vi "PSU_VOUT_Converter.vi"(0 "Output %":dbl) -> (1 "decimal integer string":string, 2 "Output % duplicate":dbl)   [LabVIEW 2022 SP3]
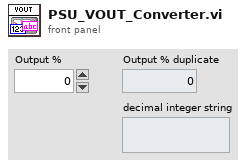
[diagram p1: front panel]
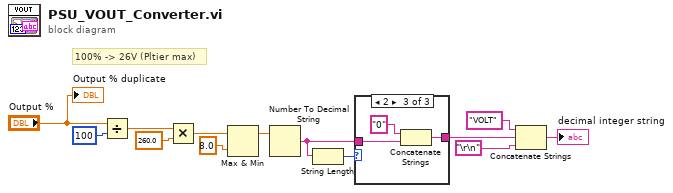
[diagram p0: block diagram]
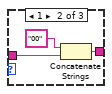
[diagram p3: hidden frame]
diagram:
  # "100% -> 26V (Pltier max)"
  n1 = Divide(x="Output %", y=100) -> (x/y=w12:dbl)
  n2 = Multiply(x=w12, y=260.0 ("x")) -> (x*y=w7:dbl)
  n3 = Max & Min(x=w7, y=8.0 ("x")) -> (max(x,y)=w5:dbl)  [unwired: 1 out]
  n4 = Number To Decimal String(number=w5) -> (decimal integer string=w2:string)  [unwired: 1 in]
  n5 = String Length(string=w2) -> (length=w4:i32)
  n6 = case shown="2" w4 {
    tunnel: [w14 w16 w19] -> w3
    tunnel: w2 -> [w14 w17 w20]
    frame 0, Default {
    }
    frame 1 {
      n7 = Concatenate Strings("00" ("string"), w17) -> (w16:string)
    }
    frame 2 {
      n8 = Concatenate Strings("0" ("string"), w20) -> (w19:string)
    }
  }
  n9 = Concatenate Strings("VOLT" ("string"), w3, "\r\n") -> (→"decimal integer string":string)
  "Output % duplicate" <- "Output %"
